vi "Search 1DElinAll2D.vi"(8 "Source":i64[][](array[numeric]), 11 "This Array":i64[](array[numeric])) -> (3 "Match array":i32[](array[numeric]))   [LabVIEW 2023]
panel:
  out "idx":i32
  out "Row":i32
  out "Cnt match":i32
  out "This Num":string
  out "Indicator":i64[][](array[numeric])
  # "Търси всеки елемент на 1D във всеки ред на 2D."
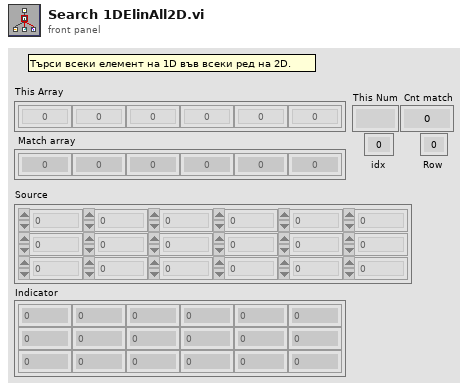
[diagram p1: front panel]
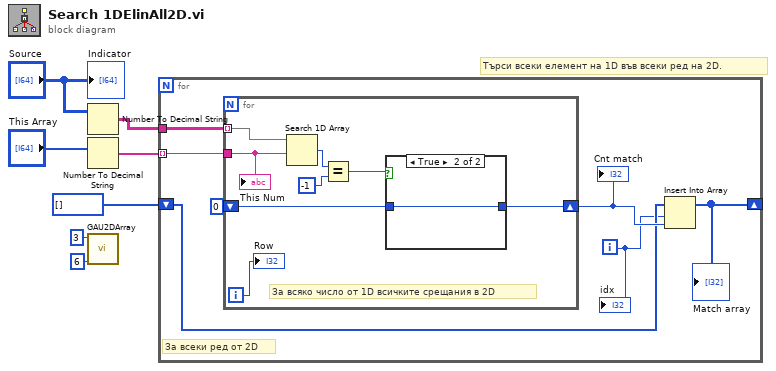
[diagram p0: block diagram]
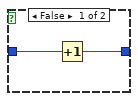
[diagram p2: hidden frame]
diagram:
  # "Търси всеки елемент на 1D във всеки ред на 2D."
  n1 = Number To Decimal String(number="Source") -> (decimal integer string=w3:string[][])  [unwired: 1 in]
  n2 = Number To Decimal String(number="This Array") -> (decimal integer string=w4:string[])  [unwired: 1 in]
  n3 = call "GAU2DArray.vi"("Colums"=6 ("Colum"), "Rows"=3 ("Row")) -> ()  [unwired: 8 in, 2 out]
  n4 = for {
    tunnel: w3 -> [w14]
    tunnel: w4 -> [w13] mode=indexing
    shift-right: [w9] -> _
    shift-left: i32[] [] -> [w10]
    i -> [w8]
    # "За всеки ред от 2D"
    n5 = for {
      tunnel: w14 -> [w22] mode=indexing
      tunnel: w13 -> [w21]
      shift-right: [w16] -> w11
      shift-left: 0 -> [w17]
      i -> [w15]
      # "За всяко число от 1D всичките срещания в 2D"
      n6 = Search 1D Array(1D array=w22, element=w21) -> (index of element=w20:i32)  [unwired: 1 in]
      n7 = Equal?(x=w20, y=-1) -> (x = y?=w18:bool)
      n8 = case shown="True" w18 {
        tunnel: w17 -> [w24 w25]
        tunnel: [w23 w25] -> w16
        frame False {
          n9 = Increment(x=w24) -> (x+1=w23:i32)
        }
        frame True {
        }
      }
      "This Num" <- w21
      "Row" <- w15
    }
    "Cnt match" <- w11
    n10 = Insert Into Array(array=w10, index=w8, new element=w11) -> (w9:i32[])
    "Match array" <- w9
    "idx" <- w8
  }
  "Indicator" <- "Source"
